vi "실습 2-1 Sine연산.vi"() -> ()   [LabVIEW 2014]
panel:
  out "x = 0?":bool
  out "숫자형 4":dbl format="%#_30e"
  out "숫자형 3":dbl format="%#_30f"
  in  "숫자형":dbl
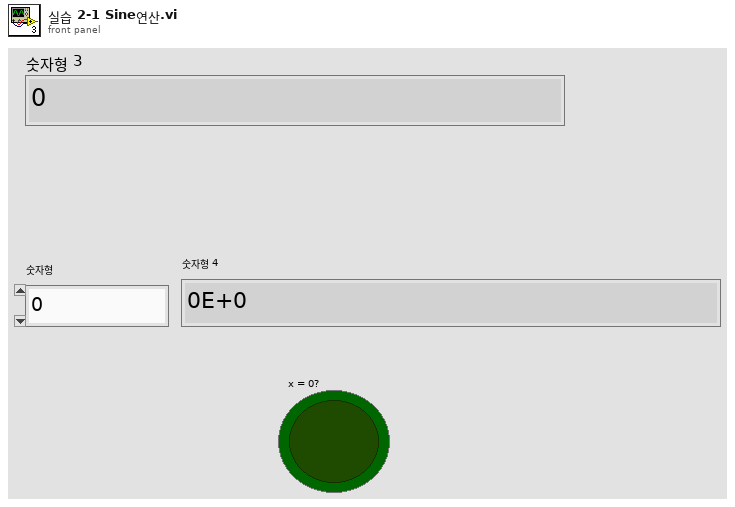
[diagram p1: front panel]
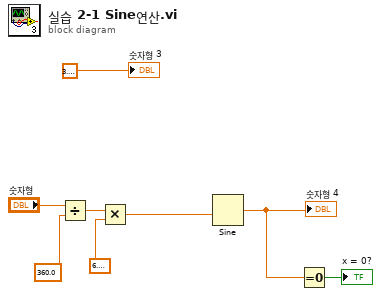
[diagram p0: block diagram]
diagram:
  n1 = Divide(x="숫자형", y=360.0) -> (x/y=w5:dbl)
  n2 = Multiply(x=w5, y=6.283185307179586) -> (x*y=w3:dbl)
  n3 = Sine(x=w3) -> (sin(x)=w2:dbl)
  "숫자형 4" <- w2
  n4 = Equal To 0?(x=w2) -> (x = 0?=→"x = 0?":bool)
  "숫자형 3" <- 3.141592653589793
